vi "Current_read_string_split.vi"(11 "String":string) -> (1 "I3":dbl, 2 "I2":dbl, 3 "I1":dbl)   [LabVIEW 2021]
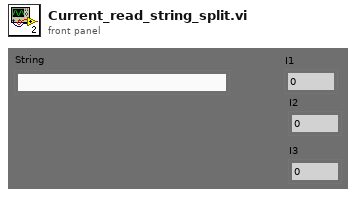
[diagram p1: front panel]
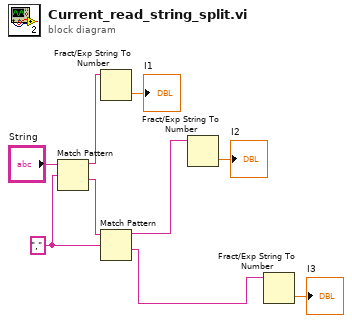
[diagram p0: block diagram]
diagram:
  w7 = "," ("regular expression")
  n1 = Match Pattern(string="String", regular expression=w7) -> (before substring=w6:string, after substring=w8:string)  [unwired: 1 in, 2 out]
  n2 = Fract/Exp String To Number(string=w6) -> (number=→"I1":dbl)  [unwired: 3 in, 1 out]
  n3 = Match Pattern(string=w8, regular expression=w7) -> (before substring=w4:string, after substring=w1:string)  [unwired: 1 in, 2 out]
  n4 = Fract/Exp String To Number(string=w4) -> (number=→"I2":dbl)  [unwired: 3 in, 1 out]
  n5 = Fract/Exp String To Number(string=w1) -> (number=→"I3":dbl)  [unwired: 3 in, 1 out]
